vi "Unserialize.vi"(6 "All Build Configs":string[](array[string]), 8 "error in (no error)":errorcluster, 9 "Serialization Version":string, 10 "XML Node":refnum<class "XML Node.lvclass">, 11 "Build Package Item in":refnum<class "VIPM Item.lvclass">) -> (0 "error out":errorcluster, 2 "Invalid Version?":bool, 3 "Build Package Item out":refnum<class "VIPM Item.lvclass">)   [LabVIEW 2019, in "VIPM.lvlib" / "VIPM Item.lvclass"]
uses:
  VIPM Item.lvclass
  libs/Solution.lvlibp/Solution/XML Reader/XML Node.lvclass
  VIPM Item.lvclass/VIPM Item.ctl
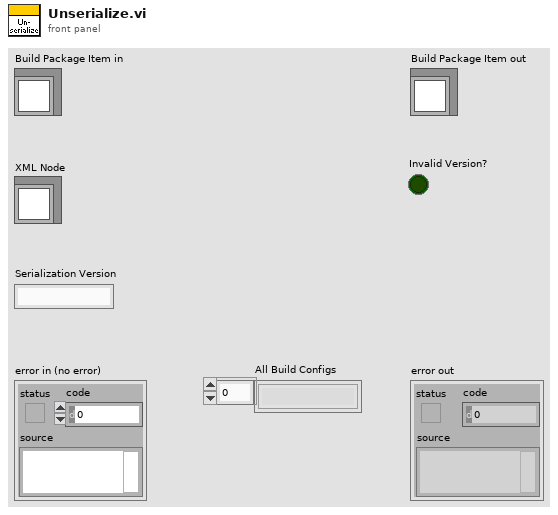
[diagram p1: front panel]
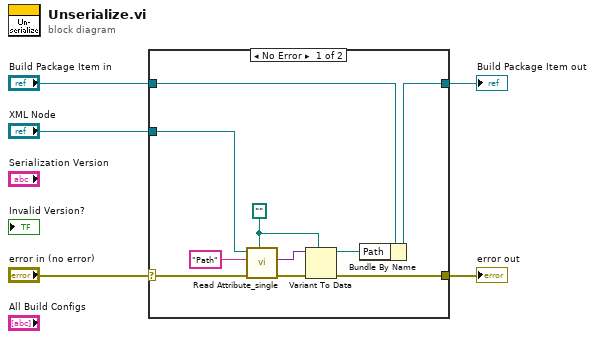
[diagram p0: block diagram]
diagram:
  n1 = case shown="No Error" "error in (no error)" {
    selector: "error in (no error)" -> [w15 w16]
    tunnel: "XML Node" -> [w12 _]
    tunnel: "Build Package Item in" -> [w11 w17]
    tunnel: [w10 w17] -> w2
    tunnel: [w9 w16] -> w1
    frame No Error {
      w7 = path ""
      n2 = call "Read Attribute_single.vi"("Type"=w7, "error in (no error)"=w15, "Name"="Path", "XML Reader in"=w12) -> ("error out"=w14:errorcluster, "Value"=w8:variant)  [unwired: 6 in]
      n3 = Variant To Data(error in=w14, type=w7, Variant=w8) -> (data=w6:path, error out=w9:errorcluster)
      n4 = Bundle By Name(cluster=w11, "Path"=w6) -> (w10:refnum<class "VIPM Item.lvclass">)
    }
    frame Error {
    }
  }
  "error out" <- w1
  "Build Package Item out" <- w2
